vi "Move Cursor into ROI.vi"(11 "Base Graph in":refnum<class "Base Graph.lvclass">) -> (3 "Base Graph out":refnum<class "Base Graph.lvclass">)   [LabVIEW 2023, in "Base Graph.lvclass"]
uses:
  Base Graph.lvclass
  Base Graph.lvclass/Base Graph.ctl
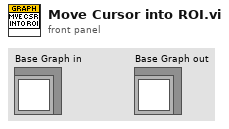
[diagram p1: front panel]
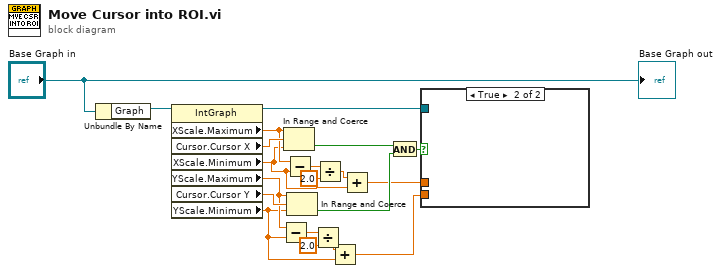
[diagram p0: block diagram]
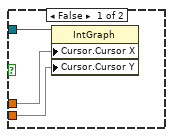
[diagram p2: hidden frame]
diagram:
  n1 = Unbundle By Name("Base Graph in") -> ("Graph"=w19:refnum<vi>)
  n2 = property class="IntGraph"(reference=w19) -> (reference out=w15:refnum<vi>, "XScale.Maximum"=w17:dbl, "Cursor.Cursor X"=w18:dbl, "XScale.Minimum"=w6:dbl, "YScale.Maximum"=w12:dbl, "Cursor.Cursor Y"=w13:dbl, "YScale.Minimum"=w9:dbl)  [unwired: 1 in, 1 out]
  n3 = Subtract(x=w12, y=w9) -> (x-y=w11:dbl)
  n4 = In Range and Coerce(upper limit=w17, x=w18, lower limit=w6) -> (In Range?=w3:bool)  [unwired: 1 out]
  n5 = Subtract(x=w17, y=w6) -> (x-y=w14:dbl)
  n6 = In Range and Coerce(upper limit=w12, x=w13, lower limit=w9) -> (In Range?=w4:bool)  [unwired: 1 out]
  n7 = Divide(x=w11, y=2.0) -> (x/y=w8:dbl)
  n8 = Divide(x=w14, y=2.0) -> (x/y=w7:dbl)
  n9 = Add(x=w8, y=w9) -> (x+y=w1:dbl)
  n10 = Add(x=w7, y=w6) -> (x+y=w2:dbl)
  n11 = And(x=w3, y=w4) -> (x .and. y?=w5:bool)
  n12 = case shown="True" w5 {
    tunnel: w15 -> [w23 _]
    tunnel: w2 -> [w22 _]
    tunnel: w1 -> [w21 _]
    frame False {
      n13 = property class="IntGraph"(reference=w23, "Cursor.Cursor X"=w22, "Cursor.Cursor Y"=w21) -> ()  [unwired: 1 in, 2 out]
    }
    frame True {
    }
  }
  "Base Graph out" <- "Base Graph in"
